vi "dvp Vi Get Color Temperature.vi"(10 "pColorTemperature":i32, 11 "handle":u32) -> (2 "pColorTemperature out":i32, 3 "function return":u32(ring))   [LabVIEW 2018, in "LabViewDVPCamera.lvlib"]
doc: "LabviewDvp2Api dvpStatus dvpViGetColorTemperature(dvpHandle handle, dvpInt32 *pColorTemperature);"
uses:
  LabViewDVPCamera.lvlib
  LabViewDVPCamera/LabViewDVPCamera.dll
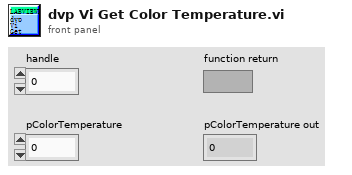
[diagram p1: front panel]
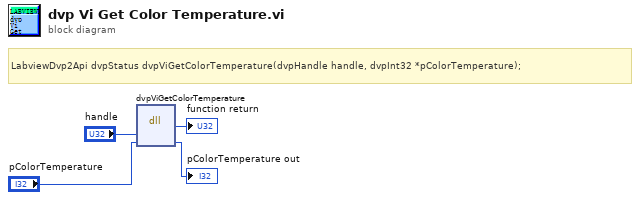
[diagram p0: block diagram]
diagram:
  # "LabviewDvp2Api dvpStatus dvpViGetColorTemperature(dvpHandle handle, dvpInt32 *pColorTemperature);"
  n1 = dll-call lib="C:/Program Files (x86)/DVP2 Labview cn 64/Sample/LabViewDVPCamera/LabViewDVPCamera.*" fn="dvpViGetColorTemperature"("handle"="handle", "pColorTemperature"="pColorTemperature") -> (→"function return":u32, "pColorTemperature"=→"pColorTemperature out":i32)  [unwired: 4 in, 2 out]
